vi "Main.vi"(8 "error in (no error)":errorcluster, 11 "Startup Notifier":refnum<notifier>) -> ()   [LabVIEW 2016, in "AssertEngine.lvlib"]
uses:
  AssertEngine/AssertEngine.lvlib
  AssertEngine/AssertEngine/AssertEngine.lvclass
  C:/Program Files/National Instruments/LabVIEW 2016/vi.lib/ActorFramework/Actor/Actor.lvclass
  <vilib>/ActorFramework/Actor/Actor.lvclass
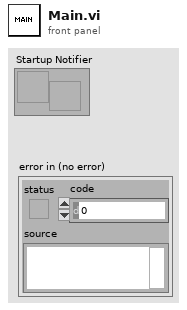
[diagram p1: front panel]
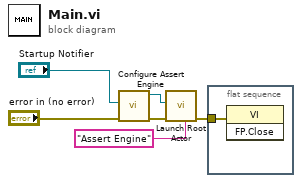
[diagram p0: block diagram]
diagram:
  n1 = call "Configure Assert Engine.vi"("error in (no error)"="error in (no error)", "Startup Notifier"="Startup Notifier") -> ("error out"=w3:errorcluster, "AssertEngine out"=w2:refnum<class "AssertEngine.lvclass">)  [unwired: 8 in]
  n2 = call <vilib>:"Launch Root Actor.vi"("Debug Alias"="Assert Engine", "error in (no error)"=w3, "Actor"=w2) -> ("error out"=w5:errorcluster)  [unwired: 7 in, 1 out]
  n3 = flat-sequence {
    tunnel: w5 -> [w7]
    frame #0 {
      n4 = invoke class="VI" method="FP.Close"(error in=w7) -> ()  [unwired: 2 in, 3 out]
    }
  }
